vi "Xml_Change_Tag_Value.vi"(7 "Tag Name":string="Spectrum_Name", 8 "error in (no error)":errorcluster, 9 "XML Filename":string="2017_03_03_018.B00.xml", 10 "XML Path":path=path "D:/PIRENEA/DATA/2017/data_2017_03_03", 11 "New Value":string="2017_03_03_018.B00.xml") -> (0 "error out":errorcluster, 2 "XML String Out":string, 3 "Old Value":string)   [LabVIEW 2018]
uses:
  <vilib>/NI/GXML/GXML.lvlib
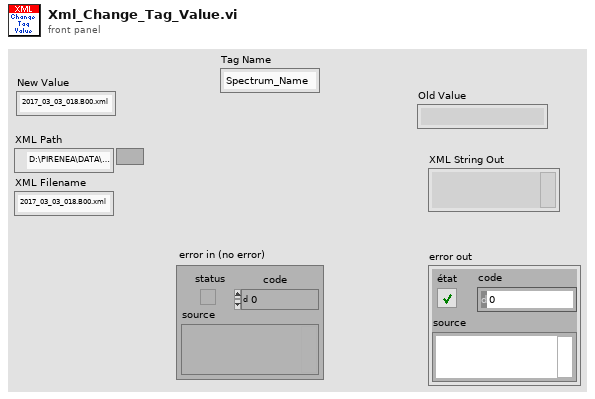
[diagram p1: front panel]
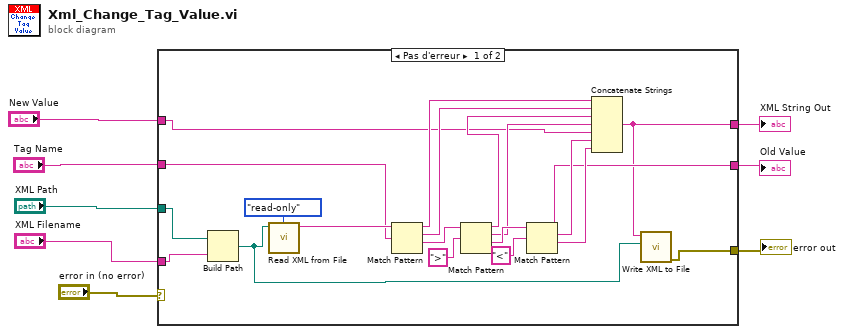
[diagram p0: block diagram]
diagram:
  n1 = case shown="Pas d'erreur" "error in (no error)" {
    selector: "error in (no error)" -> [_ w29]
    tunnel: [w11 w29] -> w7
    tunnel: "XML Path" -> [w14 _]
    tunnel: [w17 _] -> w5
    tunnel: [w12 _] -> w4
    tunnel: "XML Filename" -> [w15 _]
    tunnel: "New Value" -> [w9 _]
    tunnel: "Tag Name" -> [w10 _]
    frame No Error {
      n2 = Build Path(base path=w14, name or relative path=w15) -> (appended path=w13:path)
      n3 = call <vilib>:"Read XML from File.vi"("file access"=enum16{"read/write", "read-only", "write-only"}."read-only", "XML File Path"=w13) -> ("XML String Out"=w27:string)  [unwired: 8 in, 1 out]
      n4 = Match Pattern(string=w27, regular expression=w10) -> (before substring=w23:string, match substring=w22:string, after substring=w16:string)  [unwired: 1 in, 1 out]
      n5 = Match Pattern(string=w16, regular expression=">" ("expression régulière")) -> (before substring=w21:string, match substring=w20:string, after substring=w25:string)  [unwired: 1 in, 1 out]
      n6 = Match Pattern(string=w25, regular expression="<" ("expression régulière")) -> (before substring=w17:string, match substring=w18:string, after substring=w19:string)  [unwired: 1 in, 1 out]
      n7 = Concatenate Strings(w23, w22, w21, w20, w9, w18, w19) -> (w12:string)
      n8 = call <vilib>:"Write XML to File.vi"("XML File Path"=w13, "XML Input"=w12) -> ("error out"=w11:errorcluster)  [unwired: 9 in]
    }
    frame Error {
    }
  }
  "error out" <- w7
  "Old Value" <- w5
  "XML String Out" <- w4
